vi "GUI_Cameras_v1.4.vi"() -> ()   [LabVIEW 2013]
uses:
  <vilib>/vision/NI_Vision_Development_Module.lvlib
  shared programs/MySQL/Preset Query Enum.ctl
  color tables/image color table presets.ctl
  <vilib>/Utility/miscctls.llb/LVRectTypeDef.ctl
panel:
  in  "resize":bool
  in  "Tab Control":T1(tab)
  in  "size 2":cluster{"xhair size":dbl, "xhair size 2":dbl}={"xhair size"=20.0, "xhair size 2"=20.0} {"xhair size 2" min=0.0 max=0.0; "xhair size" min=0.0 max=0.0}
  in  "Target.X":dbl caption="TargetX"
  in  "Target.Y":dbl caption="TargetY"
  in  "draw Xhair":bool
  out "Max Counts":dbl(slide) scale=0.0..256.0
  in  "triggerdelay":dbl
  in  "trigger":bool
  in  "save":bool
  in  "exposure":dbl=0.52 caption="Exposure"
  in  "gain":dbl
  in  "shotnumber":i32=354
  in  "LowPass":bool
  in  "Size & Tolerance":T2={"X Size"=5, "Y Size"=5, "% Tolerance"=100}
  in  "LowPass":bool
  in  "Color table":T3=enum."BWR enhance low"
  in  "ROI.OffsetY":dbl
  in  "ROI.OffsetX":dbl
  in  "ROI.Height":dbl
  in  "ROI.Width":dbl
  in  "MaxGUIPixel":dbl
  out "Centroid":cluster{"X Centroid":sgl, "Y Centroid":sgl} {"Y Centroid" format="%.2f"; "X Centroid" format="%.2f"}
  out "Y Resolution":i32
  out "X Resolution":i32
  out "Mean Value":sgl format="%.2f"
  out "GUIBinning":dbl
  in  "Maximize!!":bool
  in  "LogArray":bool
  in  "hide controls":bool
  in  "sat level":sgl=255.0
  in  "beep if sat.":bool
  out "Mean Value 2":sgl(graph)
  out "histogram":T4(graph)
  out "lineout":cluster{"x0":sgl, "dx":sgl, "Pixels Line":sgl[]}(graph)
  out "MaxCounts":dbl
  in  "FWHMx":dbl
  in  "FWHMy":dbl
  out "MeanCounts":dbl
  out "FWHMx (um)":dbl
  out "FWHMy (um)":dbl
  in  "SpatialCalibration":dbl
  in  "Analysis":bool
  out "analysis error":errorcluster
  out "top":i16
  out "left":i16
  out "Zoom changed":bool
  out "Zoom old":cluster{"X":sgl, "Y":sgl}
  out "ratio(h)":bool=TRUE
  out "fixsize":bool
  out "Change Ratio":cluster{"X":sgl, "Y":sgl}={"X"=1.6671598, "Y"=0.6151203}
  out "old Panel Bounds":T5={"Left"=105, "Top"=80, "Right"=781, "Bottom"=662}
  out "error (h)":bool
  in  "Main Tap":enum32{"IMAQ", "Network", "Internal", "Array"}(tab)
  out "Image (IMAQ)":T6(plugin-control)
  out "local Port":u16=65401
  out "Remote Host":string="192.168.10.157"
  out "port or service name":u16=65400
  in  "timeout ms (slow resp)":i32=500
  in  "reset":bool
  out "All Devices (h)":string[](array[string])
  out "centroidy":dbl
  out "fast ID (h)":refnum<k16>
  out "slow ID (h)":refnum<k16>
  out "error out":errorcluster
  out "connections (hidden)":variant[](array[variant])=[variant(refnum<k16> refnum), variant(refnum<k16> refnum)]
  in  "time to wait (main loop)":i32=200
  in  "time to wait (TCP)":i32=10
  out "Data String":string="exposure,0.520000\r\ntrigger,off\r\nsave,off\r\ngain,0.000000\r\n"
  in  "send":bool
  in  "localsavingpath":path
  out "centroidy":dbl
  out "Image (array)":dbl[][](graph)
  out "Device Name (h)":string="FakeCam1"
  out "stop":bool
  out "error message":string
  out "image connection":bool
  out "data connection ok":bool
  # "Crosshair"
  # "Data"
  # "Image"
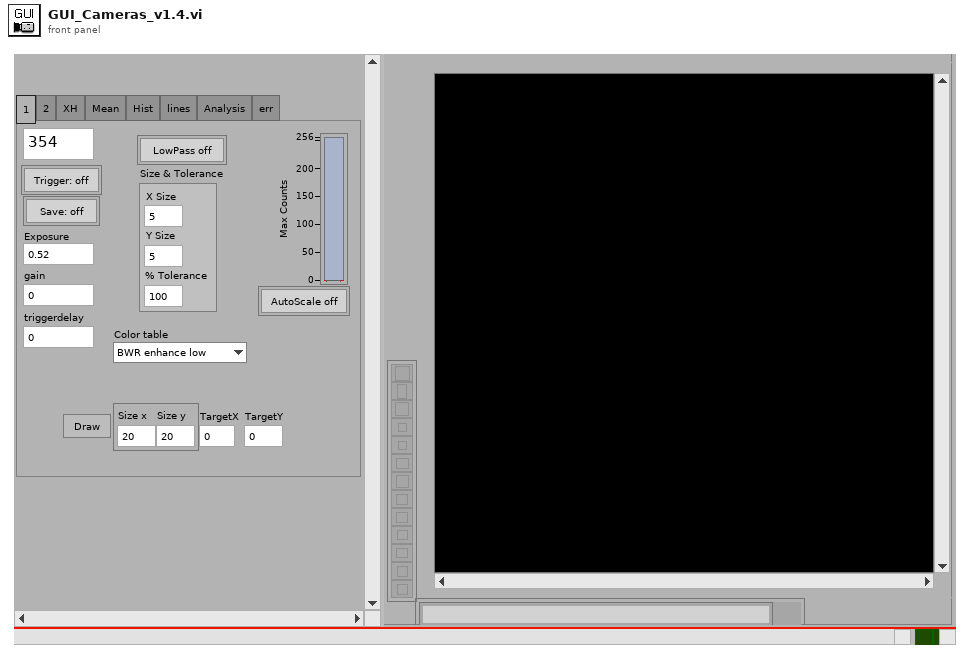
[diagram p1: front panel]
types:
  T1 = enum32{"1", "2", "XH", "Mean", "Hist", "lines", "Analysis", "err"}
  T2 = cluster{"X Size":i32, "Y Size":i32, "% Tolerance":i32}
  T3 = typedef "image color table presets.ctl" = enum16{"Greyscale", "Binary", "Gradient", "Rainbow", "Temperature", "enhance low", "blue yellow red", "BYR enhance low", "white blue yellow", "BWR enhance low", "make a new one"}
  T4 = cluster{"Starting Value":sgl, "Incremental Value":sgl, "Histogram":u32[]}
  T5 = typedef "LVRectTypeDef.ctl" = cluster{"Left":i16, "Top":i16, "Right":i16, "Bottom":i16}
  T6 = typedef "IMAQ Image.ctl" = refnum<image>
  T7 = enum16{"Grayscale", "Binary", "Gradient", "Rainbow", "Temperature", "User Defined"}
  T8 = typedef "Preset Query Enum.ctl" = enum16{"Get Locations", "Get all IPs and MACs", "Get classes", "Get expt variables to set at scanstart for particular device", "Get expt devices and variables with start values", "Get expt devices and variables (with data to get)", "Get expt devices with data to get", "Get Expt devices and GUIs", "Get all devices basic properties", "Get Virtual Devices Core Info", "Get Expt names", "Get experiment basic properties", "Get experiment alarm variables", "Get MC Ports", "Get device network comm port", "Get devicetype lvclass path", "Get basic device properties", "Get Init Order", "Get all setable variables of a device", "Get device variable aliases", "Get force values of all settable variables", "Get all variables of a devicetype", "Get all variables of a device", "Get plotter details", "Get Saved Scans", "Get Scan Info", "GetGeneralGUIs", "Get expt for plotter", "Get plotter IDs from expt", "Get all devices", "Get all Virtual Devices", "Get variable and device info for Virtual Device", "GetItemLocatorIP", "Get IPs for GUIs", "Get DeviceType from Device", "GetLocalPortRange", "GetDevicePresetVariables", "Get Device Configuration", "GetAllPresetNames", "GetAllConfigurationNames", "GetPresetDeviceNames"}
  T9 = cluster{"Left":i32, "Top":i32, "Right":i32, "Bottom":i32}
  T10 = enum32{"Invalid", "Standard", "Closed", "Hidden", "Minimized", "Maximized"}
  T11 = typedef "Image Type" = u32
  T12 = cluster{"Global Rectangle":i32[], "Contours":cluster{"Contour Type":u32, "ROI Type":u32, "Points":i32[]}[]}
  T13 = typedef "EventTypDef.ctl" = refnum<user-event>
  T14 = typedef "LVBoundsTypeDef.ctl" = cluster{"Width":u32, "Height":u32}
  T15 = typedef "ROI Descriptor" = cluster{"Global Rectangle":i32[], "Contours":cluster{"ID":enum32{"External", "Internal"}, "Type":u32, "Coordinates":i32[]}[]}
  T16 = typedef "IMAQ Line" = cluster{"Start X":i32, "Start Y":i32, "End X":i32, "End Y":i32}
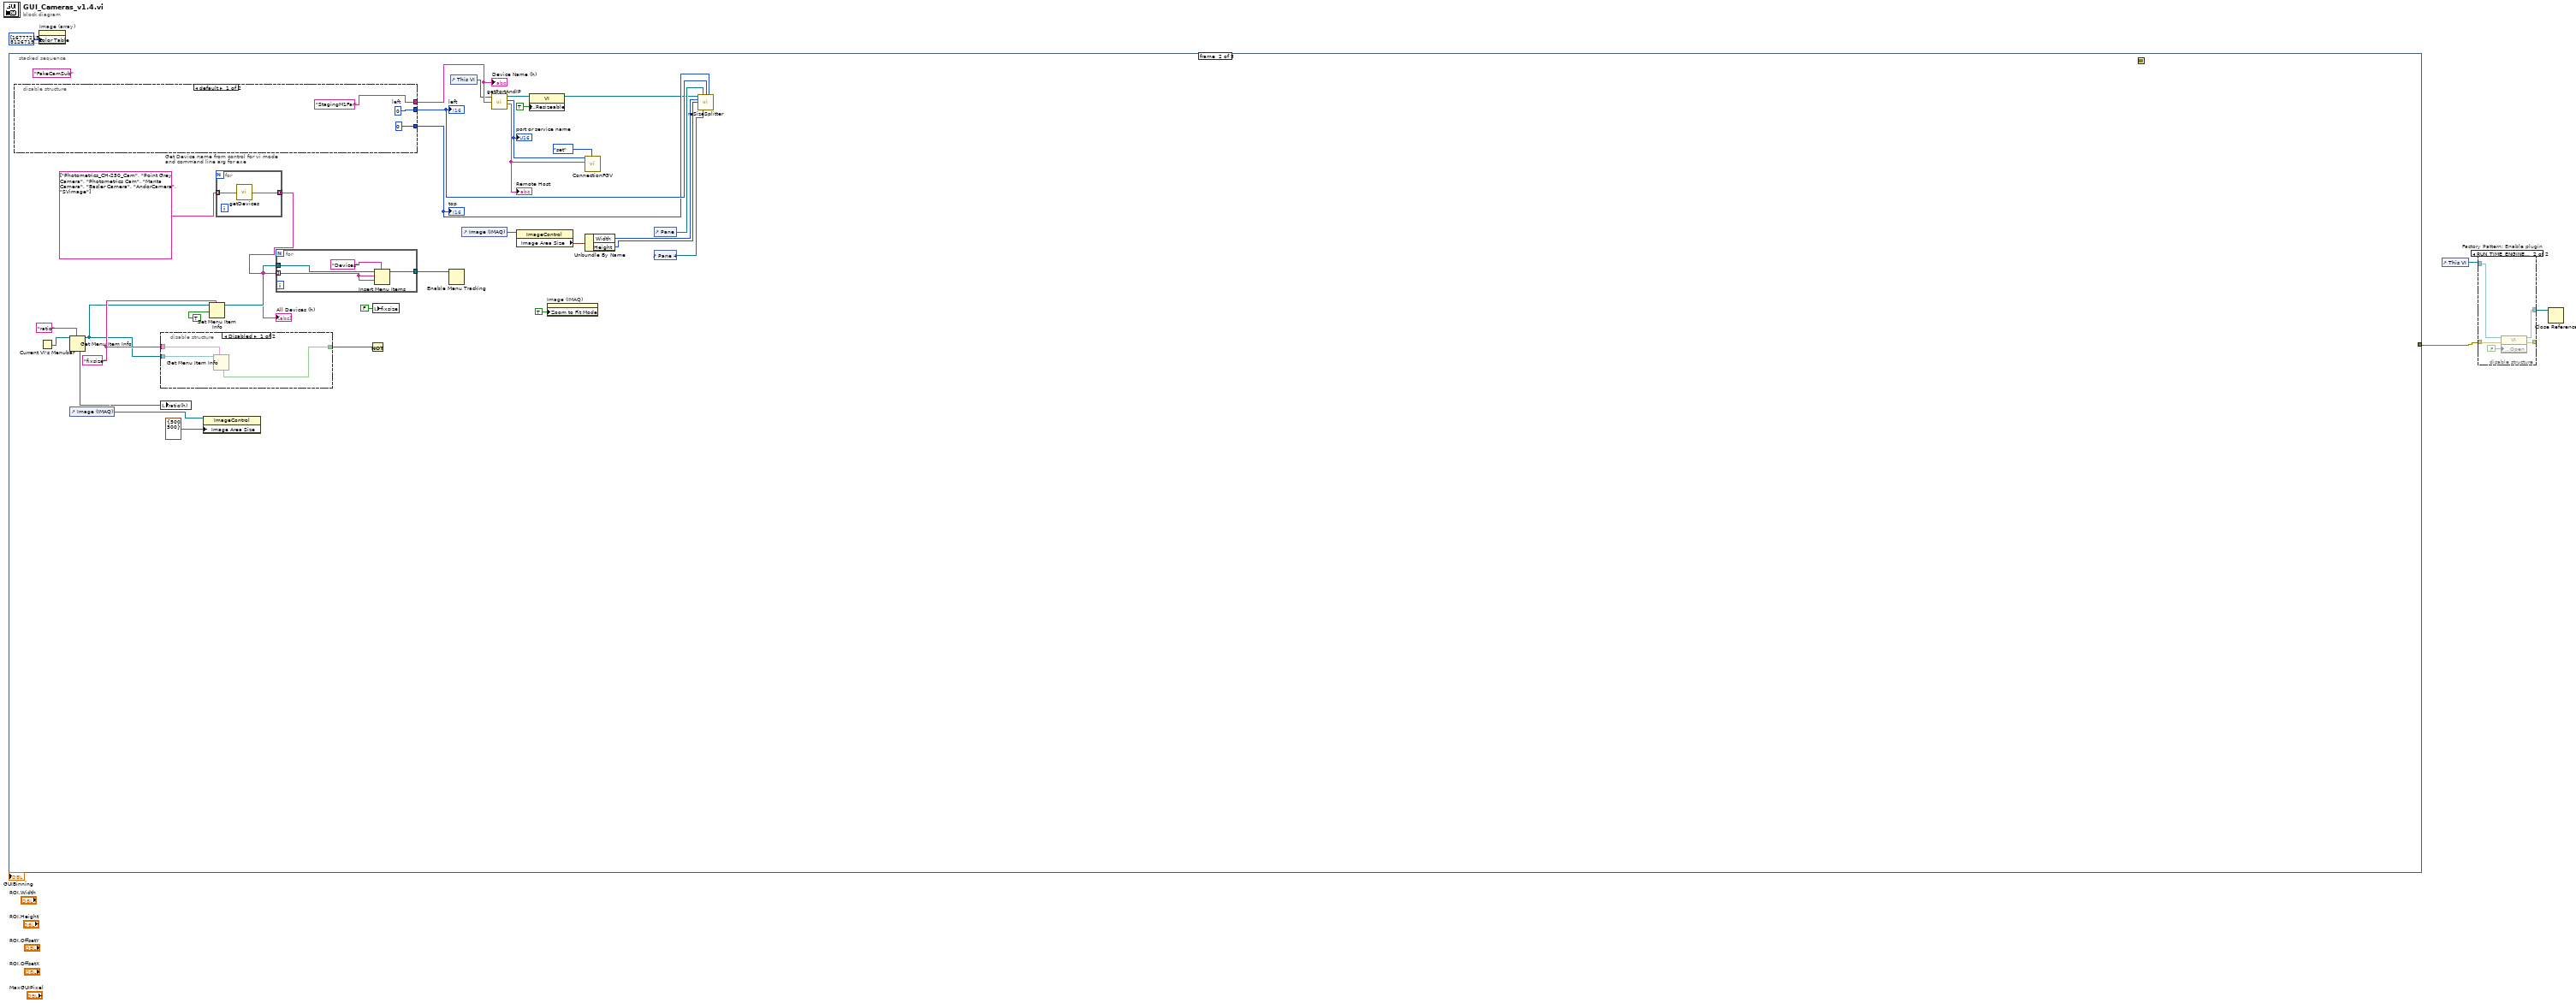
[diagram p0: block diagram]
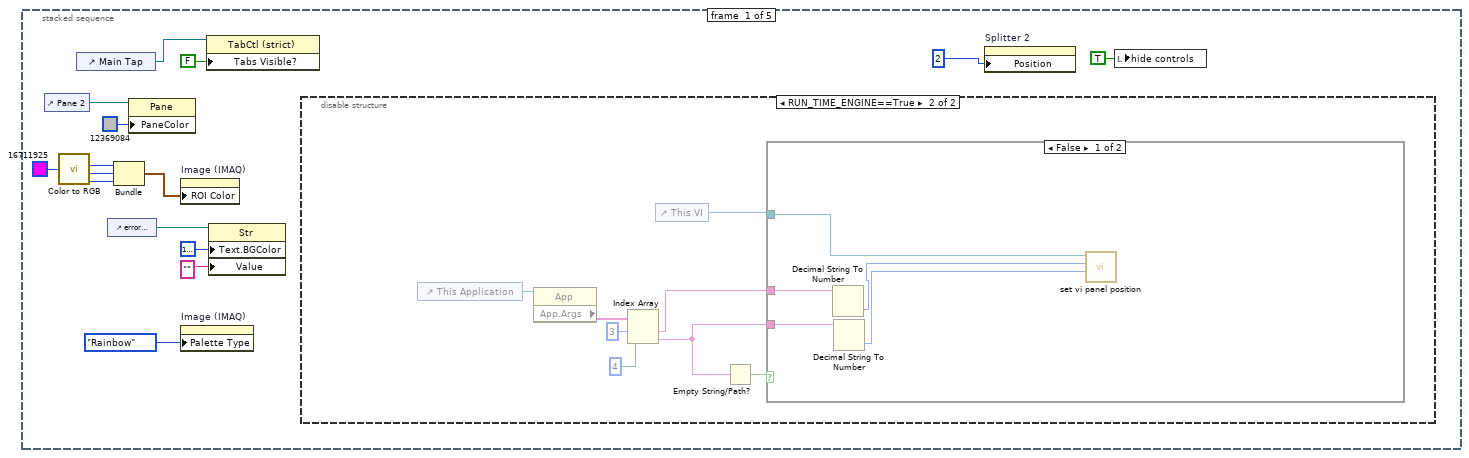
[diagram p3: hidden frame]
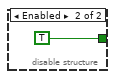
[diagram p6: hidden frame]
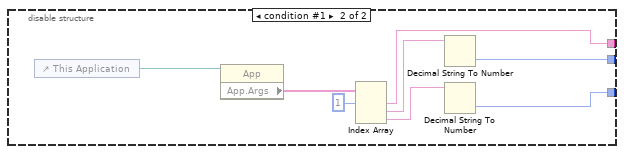
[diagram p7: hidden frame]
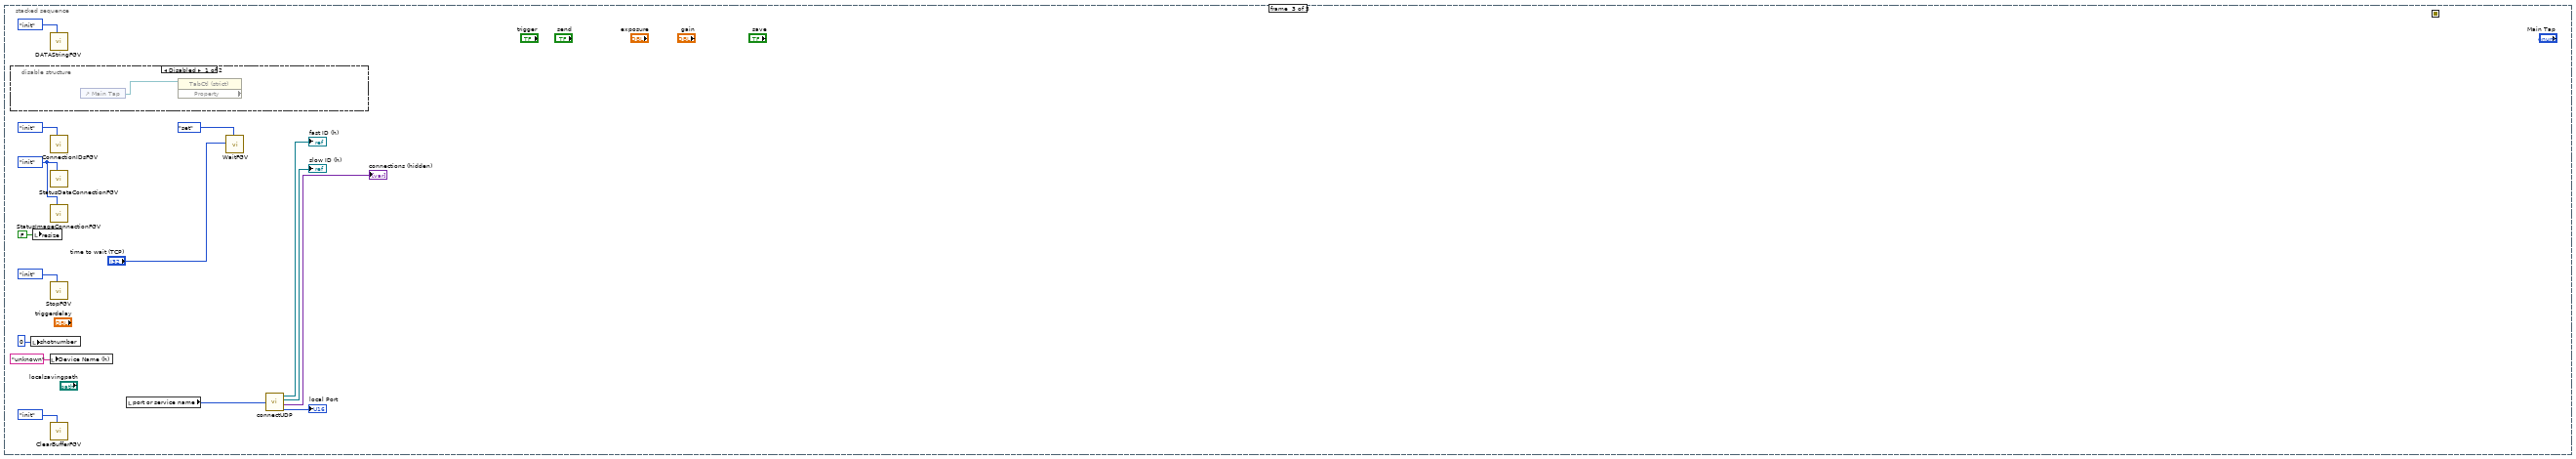
[diagram p8: hidden frame]
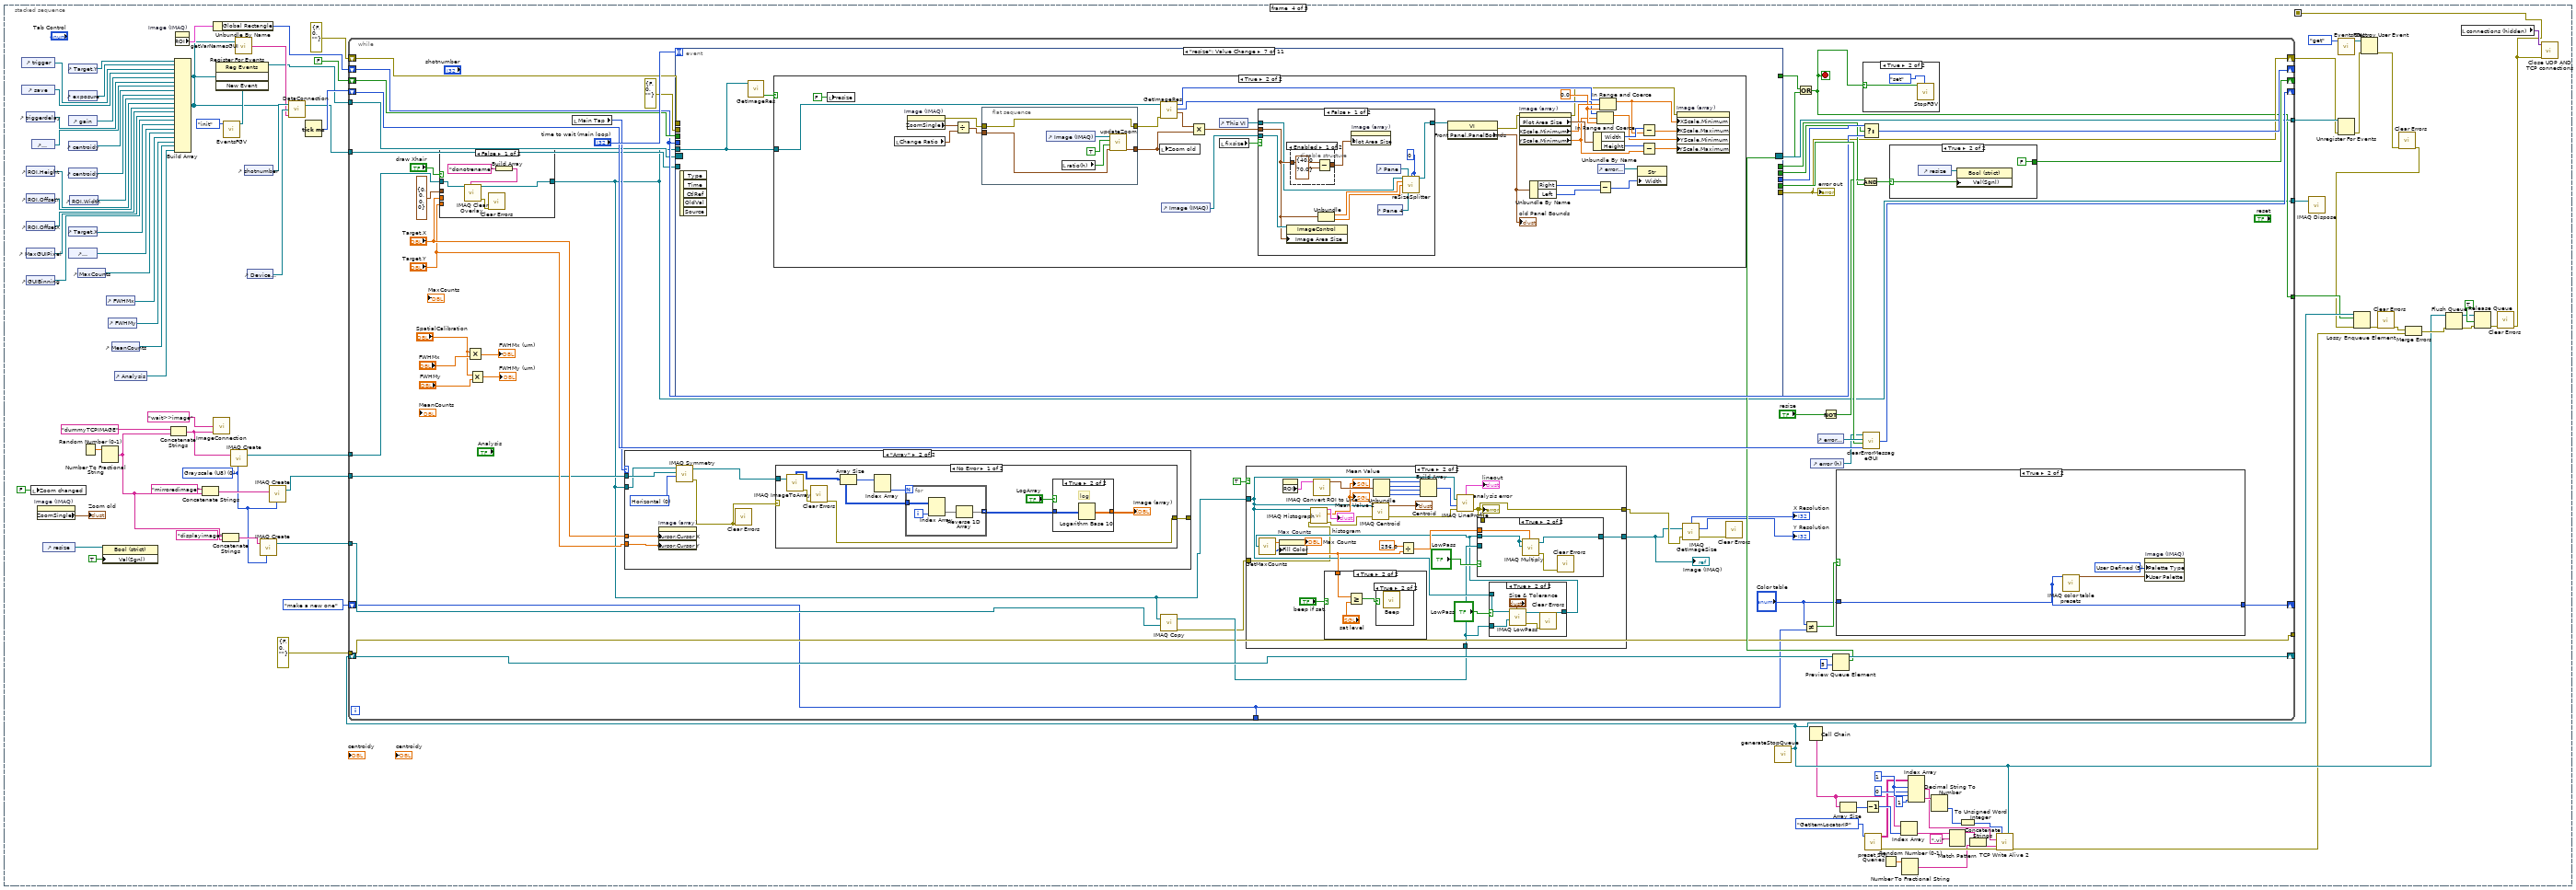
[diagram p10: hidden frame]
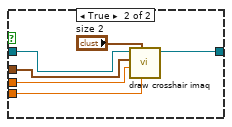
[diagram p17: hidden frame]
diagram:
  n1 = stacked-sequence {
    seq-local: [_ _ _ w135 _] -> [_ _ _ _ w558]
    tunnel: [_ _ _ _ w558] -> w2
    frame #0 {
      n2 = control-ref of="Pane 2"() -> (w14:refnum<vi>)
      n3 = call <vilib>:"Color to RGB.vi"("Color"=u32 16711925) -> ("R"=w10:u8, "G"=w9:u8, "B"=w8:u8)  [unwired: 1 out]
      n4 = control-ref of="Main Tap"() -> (w19:refnum<vi>)
      n5 = control-ref of="error message"() -> (w16:refnum<vi>)
      n6 = Bundle("R"=w10, "G"=w9, "B"=w8) -> (w7:cluster{"R":u8, "G":u8, "B":u8})  [unwired: 1 in]
      n7 = property class="Pane"(reference=w14, "PaneColor"=u32 12369084) -> ()  [unwired: 1 in, 2 out]
      n8 = property on="Image (IMAQ)" class="ImageControl"("ROI Color"=w7) -> ()  [unwired: 2 in, 2 out]
      n9 = property on="Image (IMAQ)" class="ImageControl"("Palette Type"=T7."Rainbow" ("Palette:Palette Type")) -> ()  [unwired: 2 in, 2 out]
      n10 = property class="TabCtl (strict)"(reference=w19, "Tabs Visible?"=FALSE) -> ()  [unwired: 1 in, 2 out]
      n11 = property class="Str"(reference=w16, "Text.BGColor"=u32 16777238, "Value"="") -> ()  [unwired: 1 in, 2 out]
      n12 = disable-structure shown="RUN_TIME_ENGINE==True" {
        frame condition #0 (active) {
        }
        frame condition #1 {
          n13 = control-ref of="This Application"() -> (w20:refnum<vi>)
          n14 = property class="App"(reference=w20) -> ("App.Args"=w27:string[])  [unwired: 1 in, 2 out]
          n15 = Index Array(array=w27, index #1=3 ("index"), index #2=4 ("index")) -> (element #1=w24:string, element #2=w23:string)
          n16 = control-ref of="This VI"() -> (w21:refnum<vi>)
          n17 = Empty String/Path?(string/path=w23) -> (empty?=w22:bool)
          n18 = case shown="False" w22 {
            tunnel: w24 -> [w32 _]
            tunnel: w21 -> [w28 _]
            tunnel: w23 -> [w29 _]
            frame False {
              n19 = Decimal String To Number(string=w32) -> (number=w31:i32)  [unwired: 2 in, 1 out]
              n20 = Decimal String To Number(string=w29) -> (number=w30:i32)  [unwired: 2 in, 1 out]
              n21 = call "set vi panel position.vi"("top"=w30, "left"=w31, "This VI"=w28) -> ()  [unwired: 7 in, 2 out]
            }
            frame True {
            }
          }
        }
      }
      n22 = property on="Splitter 2" class="Splitter"("Position"=2 ("Position:Left")) -> ()  [unwired: 2 in, 2 out]
      n23 = local write "hide controls"(TRUE ("hide controls")) -> ()
    }
    frame #1 {
      (unwired) "FakeCamSub" ("Device Class")
      w40 = "fixsize" ("item tag")
      n24 = disable-structure "Get Device name from control for vi mode\nand command line arg for exe" shown="default" {
        disable-tunnel: ["StagingM1Far" ("Device Name for vi mode") w81] -> w50
        disable-tunnel: [w75 w78] -> w55
        disable-tunnel: [i16 0 ("left") w77] -> w54
        frame condition #0 (active) {
          w75 = i16 0  # left
        }
        frame condition #1 {
          n25 = control-ref of="This Application"() -> (w84:refnum<vi>)
          n26 = property class="App"(reference=w84) -> ("App.Args"=w83:string[])  [unwired: 1 in, 2 out]
          n27 = Index Array(array=w83, index #1=1 ("index")) -> (element #1=w81:string, element #2=w80:string, element #3=w79:string)  [unwired: 2 in]
          n28 = Decimal String To Number(string=w80) -> (number=w78:i32)  [unwired: 2 in, 1 out]
          n29 = Decimal String To Number(string=w79) -> (number=w77:i32)  [unwired: 2 in, 1 out]
        }
      }
      "Device Name (h)" <- w50
      "left" <- w55
      "top" <- w54
      n30 = Current VI's Menubar() -> (w57:refnum<k9>)
      n31 = control-ref of="Image (IMAQ)"() -> (w43:refnum<vi>)
      n32 = Get Menu Item Info(7:"ratio" ("item tag"), 11:w57) -> (3:w39:refnum<k9>, 4:w56:bool)  [unwired: 1 in, 5 out]
      n33 = disable-structure shown="Disabled" {
        disable-tunnel: [w68 TRUE] -> w53
        disable-tunnel: w40 -> [w67 _]
        disable-tunnel: w39 -> [w66 _]
        frame Disabled {
          n34 = Get Menu Item Info(7:w67, 11:w66) -> (4:w68:bool)  [unwired: 1 in, 6 out]
        }
        frame Enabled {
        }
      }
      n35 = local write "ratio(h)"(w56) -> ()
      n36 = property class="ImageControl"(reference=w43, "Image Area Size"=cluster{"Width":u32, "Height":u32} {"Width"=500, "Height"=500} ("Image Area:Size:All Elements")) -> ()  [unwired: 1 in, 2 out]
      n37 = Set Menu Item Info(7:w40, 9:TRUE ("enabled"), 11:w39) -> (3:w38:refnum<k9>)  [unwired: 4 in, 1 out]
      n38 = for {
        tunnel: [w65] -> w34 mode=concatenating
        tunnel: string[] ["Photometrics_CH-250_Cam", "Point Grey Camera", "Photometrics Cam", "Manta Camera", "Basler Camera", "AndorCamera", "SVimage"] -> [w64] mode=indexing
        n39 = call "getDevices.vi"("Device Class"=w64) -> ("All Devices"=w65:string[])
      }
      "All Devices (h)" <- w34
      n40 = for {
        tunnel: w38 -> [w73]
        tunnel: [w72] -> w51
        tunnel: w34 -> [w70] mode=indexing
        n41 = Insert Menu Items(5:"Devices" ("menu tag"), 7:w70, 8:w70, 9:w73) -> (3:w72:refnum<k9>)  [unwired: 2 in, 2 out]
      }
      n42 = Not(x=w53) -> ()  [unwired: 1 out]
      n43 = local write "fixsize"(FALSE ("fixsize")) -> ()
      n44 = Enable Menu Tracking(4:w51) -> ()  [unwired: 2 in, 2 out]
      n45 = control-ref of="This VI"() -> (w49:refnum<vi>)
      n46 = control-ref of="Image (IMAQ)"() -> (w63:refnum<vi>)
      n47 = call "getPortAndIP.vi"("Device Name"=w50, "This Vi"=w49) -> ("Remote Host"=w44:string, "port or service name"=w45:u16, "reference out"=w48:refnum<vi>)  [unwired: 2 in, 2 out]
      "port or service name" <- w45
      "Remote Host" <- w44
      n48 = property class="ImageControl"(reference=w63) -> ("Image Area Size"=w62:cluster{"Width":u32, "Height":u32})  [unwired: 1 in, 2 out]
      n49 = property class="VI"(reference=w48, "Front Panel.Resizeable"=TRUE ("Front Panel Window:Resizable")) -> (reference out=w47:refnum<vi>)  [unwired: 1 in, 1 out]
      n50 = property on="Image (IMAQ)" class="ImageControl"("Zoom to Fit Mode"=TRUE) -> ()  [unwired: 2 in, 2 out]
      n51 = call "ConnectionFGV.vi"("command"=enum16{"get", "set", "init"}."set", "Remote Host in"=w44, "port or service name in"=w45) -> ()  [unwired: 7 in, 2 out]
      n52 = Unbundle By Name(w62) -> ("Width"=w61:u32, "Height"=w60:u32)
      n53 = control-ref of="Pane"() -> (w59:refnum<vi>)
      n54 = control-ref of="Pane 4"() -> (w52:refnum<vi>)
      n55 = call "reSizeSplitter.vi"("this vi"=w47, "pane"=w59, "left"=w55, "top"=w54, "Width"=w61, "Height"=w60, "pane2"=w52) -> ()  [unwired: 8 in, 1 out]
    }
    frame #2 {
      w95 = enum16{"get", "set", "init"}."init" ("Command")
      n56 = disable-structure shown="Disabled" {
        frame Disabled {
          n57 = control-ref of="Main Tap"() -> (w100:refnum<vi>)
          n58 = property class="TabCtl (strict)" props=[](reference=w100) -> ()  [unwired: 1 in, 3 out]
        }
        frame Enabled {
        }
      }
      n59 = local write "shotnumber"(0 ("shotnumber")) -> ()
      n60 = local write "resize"(FALSE ("resize")) -> ()
      n61 = call "DATAStringFGV.vi"("Command"=enum16{"get", "set", "init"}."init") -> ()  [unwired: 9 in, 2 out]
      n62 = call "ConnectionIDsFGV.vi"("Command"=enum16{"add", "get", "init"}."init") -> ()  [unwired: 10 in, 1 out]
      n63 = call "StatusDataConnectionFGV.vi"("Command"=w95) -> ()  [unwired: 10 in, 1 out]
      n64 = call "StatusImageConnectionFGV.vi"("Command"=w95) -> ()  [unwired: 10 in, 1 out]
      n65 = call "StopFGV.vi"("Command"=enum16{"set", "get", "init"}."init") -> ()  [unwired: 9 in, 2 out]
      n66 = local write "Device Name (h)"("unknown" ("Device Name")) -> ()
      n67 = call "ClearBufferFGV.vi"("Command"=enum16{"set", "get", "init"}."init") -> ()  [unwired: 10 in, 1 out]
      n68 = local read "port or service name"() -> (w97:u16)
      n69 = call "WaitFGV.vi"("Command"=enum16{"get", "set", "init"}."set", "milliseconds to wait"="time to wait (TCP)") -> ()  [unwired: 9 in, 1 out]
      n70 = call "connectUDP.vi"("port or service name NOT USED"=w97) -> ("fast ID (h)"=→"fast ID (h)":refnum<k16>, "slow ID (h)"=→"slow ID (h)":refnum<k16>, "connections (hidden)"=→"connections (hidden)":variant[], "local Port"=→"local Port":u16)
    }
    frame #3 {
      w124 = 1 ("index (row)")
      w101 = T11 0 items=["Grayscale (U8)", "Grayscale (I16)", "Grayscale (SGL)", "Complex (CSG)", "RGB (U32)", "HSL (U32)", "RGB (U64)", "Grayscale (U16)"] ("Image Type")
      n71 = control-ref of="trigger"() -> (w184:refnum<vi>)
      n72 = control-ref of="save"() -> (w182:refnum<vi>)
      n73 = control-ref of="triggerdelay"() -> (w180:refnum<vi>)
      n74 = control-ref of="ROI.OffsetY"() -> (w154:refnum<vi>)
      n75 = control-ref of="ROI.OffsetX"() -> (w153:refnum<vi>)
      n76 = control-ref of="MaxGUIPixel"() -> (w152:refnum<vi>)
      n77 = control-ref of="ROI.Height"() -> (w155:refnum<vi>)
      n78 = control-ref of="GUIBinning"() -> (w151:refnum<vi>)
      n79 = local write "Zoom changed"(FALSE ("Zoom changed")) -> ()
      n80 = control-ref of="localsavingpath"() -> (w176:refnum<vi>)
      n81 = property on="Image (IMAQ)" class="ImageControl"() -> ("ZoomSingle"=→"Zoom old":cluster{"X":sgl, "Y":sgl})  [unwired: 2 in, 2 out]
      n82 = control-ref of="resize"() -> (w166:refnum<vi>)
      n83 = control-ref of="Target.Y"() -> (w149:refnum<vi>)
      n84 = control-ref of="exposure"() -> (w183:refnum<vi>)
      n85 = control-ref of="gain"() -> (w181:refnum<vi>)
      n86 = control-ref of="centroidy"() -> (w175:refnum<vi>)
      n87 = control-ref of="centroidy"() -> (w169:refnum<vi>)
      n88 = control-ref of="Target.X"() -> (w150:refnum<vi>)
      n89 = control-ref of="SpatialCalibration"() -> (w148:refnum<vi>)
      n90 = control-ref of="ROI.Width"() -> (w156:refnum<vi>)
      n91 = control-ref of="MaxCounts"() -> (w147:refnum<vi>)
      n92 = Random Number (0-1)() -> (number: 0 to 1=w189:dbl)
      n93 = Number To Fractional String(number=w189) -> (F-format string=w103:string)  [unwired: 3 in]
      n94 = property class="Bool (strict)"(reference=w166, "Val(Sgnl)"=TRUE ("Value (Signaling)")) -> ()  [unwired: 1 in, 2 out]
      n95 = control-ref of="FWHMx"() -> (w146:refnum<vi>)
      n96 = control-ref of="FWHMy"() -> (w145:refnum<vi>)
      n97 = control-ref of="MeanCounts"() -> (w144:refnum<vi>)
      n98 = control-ref of="Analysis"() -> (w143:refnum<vi>)
      n99 = Concatenate Strings("dummyTCPIMAGE" ("Image Name"), w103) -> (w187:string)
      n100 = Build Array(w149, w183, w184, w182, w181, w180, w176, w175, w169, w156, w155, w154, w153, w152, w151, w150, w148, w147, w146, w145, w144, w143) -> (w163:refnum<vi>[])
      n101 = property on="Image (IMAQ)" class="ImageControl"() -> ("ROI"=w174:T12)  [unwired: 2 in, 2 out]
      n102 = Concatenate Strings("mirroredimage" ("string"), w103) -> (w108:string)
      n103 = Unbundle By Name(w174) -> ("Global Rectangle"=w173:i32[])
      n104 = call "ImageConnection.vi"("Image Name"=w187, "Image Subscriber list"="wait>>image") -> ()  [unwired: 2 in]
      n105 = Concatenate Strings("displayimage" ("string"), w103) -> (w105:string)
      n106 = call "EventsFGV.vi"("Command"=enum16{"get", "init"}."init") -> ("New Event"=w164:T13)  [unwired: 9 in, 1 out]
      n107 = register-events(w163, w164) -> (reference out=w162:refnum<event-registration>)  [unwired: 2 in, 1 out]
      n108 = call "IMAQ Create"("Image Name"=w187, "Image Type"=w101) -> ("New Image"=w190:T6)  [unwired: 3 in, 1 out]
      n109 = call "getVarNamesGUI.vi"("Array"=w163) -> ("String"=w168:string)  [unwired: 1 in]
      n110 = control-ref of="shotnumber"() -> (w171:refnum<vi>)
      n111 = control-ref of="Device Name (h)"() -> (w170:refnum<vi>)
      n112 = call "IMAQ Create"("Image Name"=w105, "Image Type"=w101) -> ("New Image"=w104:T6)  [unwired: 3 in, 1 out]
      n113 = call "IMAQ Create"("Image Name"=w108, "Image Type"=w101) -> ("New Image"=w107:T6)  [unwired: 3 in, 1 out]
      n114 = call "DataConnection.vi"("Subscriber list"=w168, "Device Name (h)"=w170, "shotnumber"=w171) -> ()
      n115 = Tick Count (ms)() -> (millisecond timer value=w177:u32)
      n116 = call "generateStopQueue.vi"() -> ("STOP Queue out"=w118:refnum<queue>)  [unwired: 10 in, 1 out]
      n117 = while {
        shift-right: [w225] -> w159
        shift-left: errorcluster {"status"=FALSE, "code"=0, "source"=""} ("error out") -> [w245]
        tunnel: w190 -> [w224]
        tunnel: [w201] -> w191
        tunnel: w163 -> [w232]
        shift-right: [w231] -> _
        shift-left: FALSE -> [w244]
        shift-right: [w243] -> _
        shift-left: w177 -> [w242]
        shift-right: [w237] -> _
        shift-left: w173 -> [w236]
        tunnel: w162 -> [w233]
        tunnel: [w226] -> w161
        tunnel: errorcluster {"status"=FALSE, "code"=0, "source"=""} ("error out") -> [w198]
        tunnel: [w198] -> _
        tunnel: [w209] -> w115
        shift-right: [w212] -> _
        shift-left: w118 -> [w213]
        tunnel: w107 -> [w207]
        tunnel: w104 -> [w200]
        shift-right: [w196] -> _
        shift-left: image_color_table_presets."make a new one" ("Color table") -> [w195]
        tunnel: [w195] -> _
        stop <- w209 stop-if-true
        n118 = case shown="False" "draw Xhair" {
          tunnel: "Target.Y" -> [_ w299]
          tunnel: "Target.X" -> [_ w300]
          tunnel: w224 -> [w297 w303]
          tunnel: [w296 w301] -> w201
          tunnel: T9 {"Left"=0, "Top"=0, "Right"=0, "Bottom"=0} ("Bounding Rectangle") -> [_ w302]
          frame False {
            n119 = Build Array("donotrename" ("String")) -> (w293:string[])
            n120 = call "IMAQ Clear Overlay"("Groups"=w293, "Image"=w297) -> ("error out"=w295:errorcluster, "Image Out"=w296:T6)  [unwired: 8 in]
            n121 = call <vilib>:"Clear Errors.vi"("error in (no error)"=w295) -> ()  [unwired: 6 in, 1 out]
          }
          frame True {
            n122 = call "draw crosshair imaq.vi"("Target.Y"=w299, "size"="size 2", "Target.X"=w300, "Bounding Rectangle"=w302, "image in"=w303) -> ("image out"=w301:T6)  [unwired: 5 in, 1 out]
          }
        }
        n123 = Multiply(x="SpatialCalibration", y="FWHMx") -> (x*y=→"FWHMx (um)":dbl)
        n124 = Multiply(x="SpatialCalibration", y="FWHMy") -> (x*y=→"FWHMy (um)":dbl)
        n125 = local read "Main Tap"() -> (w239:enum32{"IMAQ", "Network", "Internal", "Array"})
        n126 = case shown="\"Array\"" w239 {
          tunnel: w201 -> [_ w314]
          tunnel: "Target.X" -> [_ w317]
          tunnel: "Target.Y" -> [_ w316]
          tunnel: w207 -> [_ w315]
          tunnel: [_ w310] -> _
          frame "IMAQ", Default {
          }
          frame "Array" {
            w313 = u32 0 items=["Horizontal", "Vertical", "Central", "1st Diagonal", "2nd Diagonal"] ("Type of Symmetry")
            n127 = property on="Image (array)" class="IntGraph (strict)"("Cursor.Cursor X"=w317, "Cursor.Cursor Y"=w316) -> ()  [unwired: 2 in, 2 out]
            n128 = call "IMAQ Symmetry"("Type of Symmetry"=w313, "Image Dst"=w315, "Image Src"=w314) -> ("error out"=w311:errorcluster, "Image Dst Out"=w312:T6)  [unwired: 2 in]
            n129 = call <vilib>:"Clear Errors.vi"("error in (no error)"=w311) -> ()  [unwired: 6 in, 1 out]
            n130 = case shown="No Error" w311 {
              tunnel: w312 -> [w320 _]
              tunnel: [w319 _] -> w310
              frame No Error {
                n131 = call "IMAQ ImageToArray"("Image"=w320) -> ("error out"=w326:errorcluster, "Image Pixels (U8)"=w318:u8[][])  [unwired: 3 in, 3 out]
                n132 = call <vilib>:"Clear Errors.vi"("error in (no error)"=w326) -> ("error out"=w319:errorcluster)  [unwired: 6 in]
                n133 = Array Size(array=w318) -> (size(s)=w325:i32[])
                n134 = Index Array(array=w325) -> (element #2=w324:i32)  [unwired: 2 in, 1 out]
                n135 = for {
                  N: w324 -> [_]
                  tunnel: w318 -> [w333]
                  tunnel: [w331] -> w322 mode=indexing
                  i -> [w330]
                  n136 = Index Array(array=w333, index (col)=w330) -> (element=w332:u8[])  [unwired: 1 in]
                  n137 = Reverse 1D Array(array=w332) -> (reversed array=w331:u8[])
                }
                n138 = case shown="True" "LogArray" {
                  tunnel: w322 -> [w327 w329]
                  tunnel: [w327 w328] -> w321
                  frame False {
                  }
                  frame True {
                    # "log"
                    n139 = Logarithm Base 10(1:w329) -> (0:w328:dbl[][])
                  }
                }
                "Image (array)" <- w321
              }
              frame Error {
              }
            }
          }
        }
        n140 = event shown="[6] \"resize\": Value Change" {
          selector: w233 -> [_ _ _ _ _ _ _ _ _ _ _]
          dyn-events: [_ _ _ _ _ _ _ _ _ _ _] -> w226
          timeout: "time to wait (main loop)" -> [_ _ _ _ _ _ _ _ _ _ _]
          tunnel: [w339 _ _ _ _ _ _ w457 _ _ _] -> w225
          tunnel: errorcluster {"status"=FALSE, "code"=0, "source"=""} ("error out") -> [w341 _ _ _ _ _ _ _ _ _ _]
          tunnel: w245 -> [_ _ _ _ _ _ _ w457 _ _ _]
          tunnel: [TRUE _ _ _ _ _ _ _ _ _ _] -> w240
          tunnel: [_ _ _ _ _ _ _ _ w460 _ _] -> w211
          tunnel: w244 -> [_ _ _ _ _ _ _ _ _ _ _]
          tunnel: [_ w349 w361 TRUE _ _ _ _ _ _ _] -> w228
          tunnel: [_ _ _ _ _ _ _ _ _ _ w534] -> w238
          tunnel: w236 -> [_ _ _ _ _ _ _ _ _ _ w535]
          tunnel: [_ _ _ _ _ _ _ _ _ _ w533] -> w235
          tunnel: w201 -> [_ _ _ _ _ _ w401 _ _ _ w536]
          tunnel: w232 -> [_ _ _ _ _ w391 _ _ _ _ _]
          event Value Change {
            n141 = event-data() -> ("CtlRef"=w336:refnum<vi>, "NewVal"=w335:variant)  [unwired: 1 in, 3 out]
            n142 = call "SendCommandEvent.vi"("timeout ms (slow resp)"="timeout ms (slow resp)", "error out 2"=w341, "NewVal"=w335, "CtlRef"=w336) -> ("error out"=w339:errorcluster, "error (h)"=→"error (h)":bool, "error message"=→"error message":string)  [unwired: 4 in, 1 out]
          }
          event Panel Resize {
            n143 = event-data() -> ("Time"=w347:u32, "OldBnds"=w344:T5, "NewBnds"=w343:T5)  [unwired: 1 in, 4 out]
            n144 = Tick Count (ms)() -> (millisecond timer value=w348:u32)
            n145 = Subtract(x=w348, y=w347) -> (x-y=w346:u32)
            n146 = Equal?(x=w344, y=w343) -> (x = y?=w342:bool)
            n147 = Greater?(x=w346, y=u32 1000) -> ()  [unwired: 1 out]
            n148 = case shown="True" w342 {
              tunnel: w343 -> [w355 _]
              tunnel: [TRUE _] -> w349
              tunnel: w344 -> [_ _]
              frame True {
                n149 = local read "old Panel Bounds"() -> (w350:T5)
                n150 = call "getWidthAndHight.vi"("OldBnds"=w350) -> ("output cluster"=w353:cluster{"X":sgl, "Y":sgl})
                n151 = call "getWidthAndHight.vi"("OldBnds"=w355) -> ("output cluster"=w352:cluster{"X":sgl, "Y":sgl})
                n152 = Divide(x=w353, y=w352) -> (x/y=→"Change Ratio":cluster{"X":sgl, "Y":sgl})
              }
              frame False {
              }
            }
          }
          event "Maximize!!": Value Change {
            n153 = event-data() -> ()  [unwired: 1 in, 5 out]
            n154 = property class="VI"() -> (error out=w356:errorcluster, "Front Panel.PanelBounds"=w357:T5)  [unwired: 2 in, 1 out]
            n155 = case shown="True" "Maximize!!" {
              tunnel: w357 -> [w371 w375]
              tunnel: [w371 w375] -> w359
              tunnel: [_ w374] -> w358
              tunnel: w356 -> [_ w372]
              frame False {
              }
              frame True {
                n156 = local write "Maximize!!"(FALSE ("Maximize!!")) -> ()
                n157 = property class="VI"(error in=w372, "Front Panel Window:State"=T10."Maximized") -> (error out=w374:errorcluster)  [unwired: 1 in, 1 out]
                n158 = Wait (ms)(milliseconds to wait=u32 200) -> ()  [unwired: 1 out]
              }
            }
            n159 = case shown="True" TRUE {
              tunnel: [TRUE _] -> w361
              tunnel: w359 -> [w367 _]
              tunnel: w358 -> [w365 _]
              frame True {
                n160 = property class="VI"(error in=w365) -> ("Front Panel.PanelBounds"=w366:T5)  [unwired: 1 in, 2 out]
                n161 = call "getWidthAndHight.vi"("OldBnds"=w367) -> ("output cluster"=w370:cluster{"X":sgl, "Y":sgl})
                n162 = call "getWidthAndHight.vi"("OldBnds"=w366) -> ("output cluster"=w369:cluster{"X":sgl, "Y":sgl})
                n163 = Divide(x=w370, y=w369) -> (x/y=w363:cluster{"X":sgl, "Y":sgl})
                n164 = local write "Change Ratio"(w363) -> ()
                n165 = local write "resize"(TRUE ("resize")) -> ()
              }
              frame False {
              }
            }
          }
          event "hide controls": Value Change {
            n166 = event-data() -> ("NewVal"=w381:bool)  [unwired: 1 in, 4 out]
            n167 = case shown="True" w381 {
              tunnel: [367 ("Position:Left") 2 ("Position:Left")] -> w380
              frame False {
              }
              frame True {
              }
            }
            n168 = local write "Change Ratio"(cluster{"X":sgl, "Y":sgl} {"X"=1.0, "Y"=1.0} ("Change Ratio")) -> ()
            n169 = property on="Splitter 2" class="Splitter"("Position"=w380) -> ()  [unwired: 2 in, 2 out]
          }
          event "reset": Value Change {
            n170 = event-data() -> ()  [unwired: 1 in, 5 out]
            n171 = flat-sequence {
              frame #0 {
                n172 = local read "connections (hidden)"() -> (w385:variant[])
                n173 = call "Close UDP AND TCP connections.vi"("appended array"=w385) -> ()  [unwired: 7 in]
              }
              frame #1 {
                n174 = call "ConnectionFGV.vi"("command"=enum16{"get", "set", "init"}."get") -> ("port or service name out"=w387:u16)  [unwired: 9 in, 1 out]
                n175 = call "connectUDP.vi"("port or service name NOT USED"=w387) -> ("connections (hidden)"=w386:variant[])  [unwired: 3 out]
                n176 = local write "connections (hidden)"(w386) -> ()
              }
              frame #2 {
                n177 = Wait (ms)(milliseconds to wait=u32 500) -> ()  [unwired: 1 out]
              }
              frame #3 {
                n178 = property on="Image (IMAQ)" class="ImageControl"("Zoom to Fit Mode"=TRUE) -> ()  [unwired: 2 in, 2 out]
              }
            }
            n179 = local write "reset"(FALSE ("reset")) -> ()
          }
          event User Event {
            n180 = event-data() -> ("EventEnum"=w392:enum16{"new data", "connection status update"})  [unwired: 1 in, 3 out]
            n181 = case shown="\"new data\", Default" w392 {
              tunnel: w391 -> [w394 _]
              frame "new data", Default {
                n182 = call "DATAStringFGV.vi"("Command"=enum16{"get", "set", "init"}."get") -> ("Data String out"=w393:string)  [unwired: 9 in, 1 out]
                "Data String" <- w393
                n183 = call "Update Indicators (Data String to ref array).vi"("Array"=w394, "Data String"=w393) -> ()  [unwired: 12 in, 2 out]
              }
              frame "connection status update" {
                n184 = call "StatusDataConnectionFGV.vi"("Command"=enum16{"get", "set", "init"}."get") -> ("Data Connection out"=→"image connection":bool)  [unwired: 10 in]
                n185 = call "StatusImageConnectionFGV.vi"("Command"=enum16{"get", "set", "init"}."get") -> ("Image Connection out"=→"data connection ok":bool)  [unwired: 10 in]
              }
            }
          }
          event "resize": Value Change {
            n186 = event-data() -> ()  [unwired: 1 in, 5 out]
            n187 = call "GetImageRes.vi"("Image"=w401) -> ("valid Image"=w400:bool)  [unwired: 6 in, 4 out]
            n188 = case shown="True" w400 {
              tunnel: w401 -> [_ w410]
              frame False {
                n189 = local write "resize"(FALSE ("resize")) -> ()
              }
              frame True {
                w418 = 0.0 ("lower limit")
                n190 = local write "resize"(FALSE ("resize")) -> ()
                n191 = local read "Change Ratio"() -> (w434:cluster{"X":sgl, "Y":sgl})
                n192 = property on="Image (IMAQ)" class="ImageControl"() -> (error out=w405:errorcluster, "ZoomSingle"=w435:cluster{"X":sgl, "Y":sgl})  [unwired: 2 in, 1 out]
                n193 = Divide(x=w435, y=w434) -> (x/y=w404:cluster{"X":sgl, "Y":sgl})
                n194 = flat-sequence {
                  tunnel: [w439] -> w403
                  tunnel: w404 -> [w437]
                  tunnel: [w436] -> w406
                  tunnel: w405 -> [w436]
                  frame #0 {
                    n195 = control-ref of="Image (IMAQ)"() -> (w441:refnum<vi>)
                    n196 = local read "ratio(h)"() -> (w440:bool)
                    n197 = call "updateZoom.vi"("Zoom old"=w437, "ratio(h)"=w440, "update Zoom"=TRUE, "imageRef"=w441) -> ("Zoom out"=w439:cluster{"X":sgl, "Y":sgl})  [unwired: 7 in]
                  }
                }
                n198 = local write "Zoom old"(w403) -> ()
                n199 = call "GetImageRes.vi"("error in (no error)"=w406, "Image"=w410) -> ("Image Area:Size:All Elements"=w411:cluster{"Width":u32, "Height":u32}, "Y Resolution"=w412:i32, "X Resolution"=w413:i32)  [unwired: 5 in, 2 out]
                n200 = control-ref of="Image (IMAQ)"() -> (w425:refnum<vi>)
                n201 = Multiply(x=w411, y=w403) -> (x*y=w433:cluster{sgl, sgl})
                n202 = control-ref of="This VI"() -> (w414:refnum<vi>)
                n203 = local read "fixsize"() -> (w426:bool)
                n204 = case shown="False" w426 {
                  tunnel: w433 -> [w445 _]
                  tunnel: w414 -> [w442 w456]
                  tunnel: [w448 w456] -> w431
                  tunnel: w425 -> [w447 _]
                  frame False {
                    w443 = i16 0 ("left")
                    n205 = property class="ImageControl"(reference=w447, "Image Area Size"=w445) -> ()  [unwired: 1 in, 2 out]
                    n206 = disable-structure shown="Enabled" {
                      disable-tunnel: w445 -> [w454 w455]
                      disable-tunnel: [w453 w455] -> w444
                      frame Enabled {
                        n207 = Subtract(x=w454, y=cluster{sgl, sgl} {40.0, 70.0}) -> (x-y=w453:cluster{sgl, sgl})
                      }
                      frame Disabled {
                      }
                    }
                    n208 = Unbundle(w445) -> (w450:sgl, w451:sgl)
                    n209 = property on="Image (array)" class="IntGraph (strict)"("Plot Area Size"=w444) -> ()  [unwired: 2 in, 2 out]
                    n210 = control-ref of="Pane"() -> (w449:refnum<vi>)
                    n211 = control-ref of="Pane 4"() -> (w446:refnum<vi>)
                    n212 = call "reSizeSplitter.vi"("this vi"=w442, "pane"=w449, "left"=w443, "top"=w443, "Width"=w450, "Height"=w451, "pane2"=w446) -> ("reference out"=w448:refnum<vi>)  [unwired: 8 in]
                  }
                  frame True {
                  }
                }
                n213 = property class="VI"(reference=w431) -> (error out=w409:errorcluster, "Front Panel.PanelBounds"=w430:T5)  [unwired: 1 in, 1 out]
                "old Panel Bounds" <- w430
                n214 = property on="Image (array)" class="IntGraph (strict)"(error in=w409) -> (error out=w408:errorcluster, "Plot Area Size"=w424:T14, "XScale.Minimum"=w419:dbl, "YScale.Minimum"=w417:dbl)  [unwired: 1 in, 1 out]
                n215 = Unbundle By Name(w430) -> ("Right"=w429:i16, "Left"=w428:i16)
                n216 = Unbundle By Name(w424) -> ("Width"=w423:u32, "Height"=w421:u32)
                n217 = In Range and Coerce(upper limit=w412, x=w417, lower limit=w418) -> (coerced(x)=w416:dbl)  [unwired: 1 out]
                n218 = Subtract(x=w429, y=w428) -> (x-y=w427:i16)
                n219 = control-ref of="error message"() -> (w432:refnum<vi>)
                n220 = In Range and Coerce(upper limit=w413, x=w419, lower limit=w418) -> (coerced(x)=w420:dbl)  [unwired: 1 out]
                n221 = property class="Str"(reference=w432, "Width"=w427) -> ()  [unwired: 1 in, 2 out]
                n222 = Subtract(x=w423, y=w420) -> (x-y=w422:dbl)
                n223 = Subtract(x=w421, y=w417) -> (x-y=w415:dbl)
                n224 = property on="Image (array)" class="IntGraph (strict)"(error in=w408, "XScale.Minimum"=w420, "XScale.Maximum"=w422, "YScale.Minimum"=w416, "YScale.Maximum"=w415) -> ()  [unwired: 1 in, 2 out]
              }
            }
          }
          event Timeout {
            n225 = event-data() -> ()  [unwired: 1 in, 2 out]
          }
          event Menu Selection (User) {
            n226 = event-data() -> ("MenuRef"=w459:refnum<k9>, "ItemTag"=w458:string)  [unwired: 1 in, 3 out]
            n227 = case shown="\"Controls\"" w458 {
              tunnel: [_ w466] -> w460
              tunnel: w458 -> [_ w464]
              tunnel: w459 -> [_ w463]
              frame "Controls" {
                n228 = local read "hide controls"() -> (w462:bool)
                n229 = Not(x=w462) -> (.not. x?=w461:bool)
                n230 = property on="hide controls" class="Bool (strict)"("Val(Sgnl)"=w461) -> ()  [unwired: 2 in, 2 out]
              }
              frame Default {
                n231 = Equal?(x="Exit", y=w464) -> (x = y?=w466:bool)
                "stop" <- w466
                n232 = property on="Main Tap" class="TabCtl (strict)"() -> ("Value"=w468:enum32{"IMAQ", "Network", "Internal", "Array"})  [unwired: 2 in, 2 out]
                n233 = case shown="False" w466 {
                  tunnel: w468 -> [w527 _]
                  tunnel: w464 -> [w526 _]
                  tunnel: [w523 errorcluster {"status"=FALSE, "code"=0, "source"=""} ("error out")] -> w465
                  frame False {
                    n234 = call <userlib>:"Set Enum String Value__ogtk.vi"("String Value"=w526, "Default Enum Value"=w527) -> ("error out"=w525:errorcluster, "Enum"=w529:variant)  [unwired: 8 in]
                    n235 = Variant To Data(error in=w525, type=w527, Variant=w529) -> (data=w528:enum32{"IMAQ", "Network", "Internal", "Array"}, error out=w524:errorcluster)
                    n236 = property on="Main Tap" class="TabCtl (strict)"(error in=w524, "Value"=w528) -> (error out=w523:errorcluster)  [unwired: 1 in, 1 out]
                  }
                  frame True {
                  }
                }
                n237 = case shown="Error" w465 {
                  tunnel: w463 -> [_ w472]
                  tunnel: w464 -> [_ w476]
                  tunnel: [_ w477] -> _
                  frame No Error {
                  }
                  frame Error {
                    n238 = local read "All Devices (h)"() -> (w474:string[])
                    n239 = Search 1D Array(1D array=w474, element=w476) -> (index of element=w475:i32)  [unwired: 1 in]
                    n240 = Get Menu Item Info(7:w476, 11:w472) -> (0:w473:errorcluster, 2:w479:string, 4:w480:bool)  [unwired: 1 in, 4 out]
                    n241 = Not(x=w480) -> (.not. x?=w478:bool)
                    n242 = Greater Or Equal To 0?(x=w475) -> (x >= 0?=w471:bool)
                    n243 = case shown="True" w471 {
                      tunnel: w474 -> [_ w484]
                      tunnel: w473 -> [_ _]
                      tunnel: w472 -> [w481 w483]
                      tunnel: [w481 w482] -> w470
                      frame False {
                      }
                      frame True {
                        n244 = for {
                          tunnel: w484 -> [w488] mode=indexing
                          tunnel: w483 -> [w486]
                          tunnel: [w485] -> w482
                          n245 = Set Menu Item Info(6:FALSE ("checked"), 7:w488, 11:w486) -> (3:w485:refnum<k9>)  [unwired: 4 in, 1 out]
                        }
                      }
                    }
                    n246 = case shown="Default" w476 {
                      selector: w476 -> [_ w494 _ _ w515 _ _]
                      tunnel: w478 -> [w489 w492 w505 _ _ _ w520]
                      tunnel: [_ _ TRUE _ _ _ _] -> w477
                      tunnel: w471 -> [_ w495 _ _ _ _ _]
                      tunnel: [w489 w493 w505 _ _ _ w520] -> w469
                      frame "fixsize" {
                        n247 = Not(x=w489) -> (.not. x?=w490:bool)
                        n248 = control-ref of="This VI"() -> (w491:refnum<vi>)
                        n249 = property class="VI"(reference=w491, "Front Panel.Resizeable"=w490) -> ()  [unwired: 1 in, 2 out]
                        "fixsize" <- w489
                      }
                      frame Default {
                        n250 = case shown="True" w495 {
                          tunnel: w494 -> [_ w503]
                          tunnel: [_ w499] -> w493
                          tunnel: w492 -> [_ w499]
                          frame False {
                          }
                          frame True {
                            n251 = control-ref of="This VI"() -> (w502:refnum<vi>)
                            n252 = control-ref of="reset"() -> (w501:refnum<vi>)
                            n253 = call "getPortAndIP.vi"("Device Name"=w503, "This Vi"=w502) -> ("Remote Host"=w496:string, "port or service name"=w497:u16)  [unwired: 2 in, 3 out]
                            n254 = local write "port or service name"(w497) -> ()
                            n255 = local write "Remote Host"(w496) -> ()
                            n256 = property class="Bool (strict)"(reference=w501, "Val(Sgnl)"=TRUE ("Value (Signaling)")) -> ()  [unwired: 1 in, 2 out]
                            n257 = call "ConnectionFGV.vi"("command"=enum16{"get", "set", "init"}."set", "Remote Host in"=w496, "port or service name in"=w497) -> ()  [unwired: 7 in, 2 out]
                          }
                        }
                      }
                      frame "ratio" {
                        n258 = property on="Image (IMAQ)" class="ImageControl"() -> ("ZoomSingle"=w504:cluster{"X":sgl, "Y":sgl})  [unwired: 2 in, 2 out]
                        n259 = local write "Zoom old"(w504) -> ()
                        "ratio(h)" <- w505
                      }
                      frame "Local Saving Path" {
                        n260 = control-ref of="localsavingpath"() -> (w507:refnum<vi>)
                        n261 = property class="Path"(reference=w507) -> (reference out=w510:refnum<vi>, "Value"=w511:path)  [unwired: 1 in, 1 out]
                        n262 = call "changePath.vi"("Local Saving in (h)"=w511) -> ("change (h)"=w509:bool, "Local Saving out (h)"=w508:path)  [unwired: 9 in]
                        n263 = case shown="True" w509 {
                          tunnel: w510 -> [_ w513]
                          tunnel: w508 -> [_ w512]
                          frame False {
                          }
                          frame True {
                            n264 = property class="Path"(reference=w513, "Val(Sgnl)"=w512) -> ()  [unwired: 1 in, 2 out]
                          }
                        }
                      }
                      frame "Binary", "Gradient", "Grayscale", "Rainbow", "Temperature" {
                        n265 = Scan From String(input string=w515, default 1=T7."Grayscale" ("Palette:Palette Type")) -> (output 1=w514:T7)  [unwired: 3 in, 3 out]
                        n266 = property on="Image (IMAQ)" class="ImageControl"("Palette Type"=w514) -> ()  [unwired: 2 in, 2 out]
                      }
                      frame "reset" {
                        n267 = control-ref of="reset"() -> (w518:refnum<vi>)
                        n268 = property class="Bool (strict)"(reference=w518, "Val(Sgnl)"=TRUE ("Value (Signaling)")) -> ()  [unwired: 1 in, 2 out]
                      }
                      frame "clear" {
                        n269 = control-ref of="reset"() -> (w522:refnum<vi>)
                        n270 = call "ClearBufferFGV.vi"("Command"=enum16{"set", "get", "init"}."set", "clear buffer"=w520) -> ()  [unwired: 9 in, 1 out]
                        n271 = property class="Bool (strict)"(reference=w522, "Val(Sgnl)"=TRUE ("Value (Signaling)")) -> ()  [unwired: 1 in, 2 out]
                      }
                    }
                    n272 = Set Menu Item Info(6:w469, 7:w476, 10:w479, 11:w470) -> ()  [unwired: 3 in, 2 out]
                  }
                }
              }
            }
          }
          event "time to wait (TCP)": Value Change {
            n273 = event-data() -> ("NewVal"=w532:i32)  [unwired: 1 in, 4 out]
            n274 = call "WaitFGV.vi"("Command"=enum16{"get", "set", "init"}."set", "milliseconds to wait"=w532) -> ()  [unwired: 9 in, 1 out]
          }
          event "Image (IMAQ)": Mouse Up {
            n275 = event-data() -> ()  [unwired: 1 in, 5 out]
            n276 = disable-structure shown="Disabled" {
              disable-tunnel: w536 -> [w551 _]
              disable-tunnel: w535 -> [w549 _]
              disable-tunnel: [w548 _] -> w534
              disable-tunnel: [w542 _] -> w533
              frame Disabled {
                n277 = local read "Zoom old"() -> (w539:cluster{"X":sgl, "Y":sgl})
                n278 = property on="Image (IMAQ)" class="ImageControl"() -> ("ZoomSingle"=w538:cluster{"X":sgl, "Y":sgl})  [unwired: 2 in, 2 out]
                n279 = property on="Image (IMAQ)" class="ImageControl"() -> ("ROI"=w550:T12)  [unwired: 2 in, 2 out]
                n280 = Unbundle By Name(w550) -> ("Global Rectangle"=w548:i32[])
                n281 = Unbundle By Name(w538) -> ("X"=w540:sgl)
                n282 = Unbundle By Name(w539) -> ("X"=w541:sgl)
                n283 = Not Equal?(x=w549, y=w548) -> (x != y?=w552:bool[])
                n284 = Empty Array?(array=w548) -> (empty?=w547:bool)
                n285 = Not Equal?(x=w540, y=w541) -> (x != y?=w537:bool)
                "Zoom changed" <- w537
                n286 = Empty Array?(array=w549) -> (empty?=w545:bool)
                n287 = Or Array Elements(Boolean array=w552) -> (logical OR=w543:bool)
                n288 = Not(x=w547) -> (.not. x?=w546:bool)
                n289 = case shown="True" w537 {
                  tunnel: w538 -> [_ w555]
                  frame False {
                  }
                  frame True {
                    n290 = local write "Zoom old"(w555) -> ()
                  }
                }
                n291 = case shown="True" w537 {
                  selector: w537 -> [_ w553]
                  frame False {
                  }
                  frame True {
                    n292 = control-ref of="resize"() -> (w554:refnum<vi>)
                    n293 = property class="Bool (strict)"(reference=w554, "Val(Sgnl)"=w553) -> ()  [unwired: 1 in, 2 out]
                  }
                }
                n294 = And(x=w545, y=w546) -> (x .and. y?=w544:bool)
                n295 = Or(x=w543, y=w544) -> (x .or. y?=w542:bool)
                n296 = case shown="True" w542 {
                  tunnel: w551 -> [_ _]
                  tunnel: w550 -> [_ w557]
                  frame False {
                  }
                  frame True {
                    n297 = call "ROI thickener.vi"("ROI Descriptor in"=w557) -> ("ROI Descriptor out"=w556:T15)  [unwired: 1 in, 1 out]
                    n298 = property on="Image (IMAQ)" class="ImageControl"("ROI"=w556) -> ()  [unwired: 2 in, 2 out]
                  }
                }
              }
              frame Enabled {
              }
            }
          }
        }
        "error out" <- w225
        n299 = call "IMAQ Copy"("Image Dst"=w200, "Image Src"=w201) -> ("error out"=w197:errorcluster, "Image Dst Out"=w199:T6)  [unwired: 4 in]
        n300 = case shown="True" TRUE ("localanalysis") {
          tunnel: w201 -> [w252 w256]
          tunnel: [_ w263] -> w203
          tunnel: [w252 w257] -> w202
          tunnel: w199 -> [_ w255]
          tunnel: w197 -> [_ w253]
          frame False {
          }
          frame True {
            n301 = property on="Image (IMAQ)" class="ImageControl"() -> ("ROI"=w275:T12)  [unwired: 2 in, 2 out]
            n302 = call "IMAQ Histograph"("error in (no error)"=w253, "Image"=w256) -> ("error out"=w267:errorcluster, "Mean Value"=→"Mean Value" →"Mean Value 2":sgl, "Histogram Graph"=→"histogram":T4)  [unwired: 6 in, 1 out]
            n303 = call "IMAQ Convert ROI to Line"("ROI Descriptor"=w275) -> ("Line"=w274:T16)  [unwired: 8 in, 1 out]
            n304 = call "IMAQ Centroid"("error in (no error)"=w267, "Image"=w256) -> ("error out"=w277:errorcluster, "Centroid"=→"Centroid":cluster{"X Centroid":sgl, "Y Centroid":sgl})  [unwired: 2 in]
            n305 = Unbundle(w274) -> ("Start X"=w273:i32, "Start Y"=w272:i32, "End X"=w271:i32, "End Y"=w270:i32)
            n306 = Build Array(w273, w272, w271, w270) -> (w269:i32[])
            n307 = call "IMAQ LineProfile"("error in (no error)"=w277, "Line Coordinates"=w269, "Image"=w256) -> ("error out"=w263:errorcluster, "Line Graph"=→"lineout":cluster{"x0":sgl, "dx":sgl, "Pixels Line":sgl[]})  [unwired: 2 in, 2 out]
            "analysis error" <- w263
            n308 = case shown="True" "LowPass" {
              tunnel: w256 -> [_ w282]
              tunnel: [w279 w284] -> w254
              tunnel: w255 -> [w279 w281]
              frame False {
              }
              frame True {
                n309 = call "IMAQ LowPass"("Image Src"=w282, "Size & Tolerance"="Size & Tolerance", "Image Dst"=w281) -> ("Image Dst Out"=w284:T6, "error out"=w280:errorcluster)  [unwired: 4 in]
                n310 = call <vilib>:"Clear Errors.vi"("error in (no error)"=w280) -> ()  [unwired: 6 in, 1 out]
              }
            }
            n311 = call "GetMaxCounts.vi"("New Image"=w254) -> ("Maximal Value"=w260:sgl, "Color"=w261:u32)
            "Max Counts" <- w260
            n312 = property on="Max Counts" class="Slide (strict)"("Fill Color"=w261) -> ()  [unwired: 2 in, 2 out]
            n313 = case shown="True" "beep if sat." {
              tunnel: w260 -> [_ w287]
              frame False {
              }
              frame True {
                n314 = Greater Or Equal?(x=w287, y="sat level") -> (x >= y?=w285:bool)
                n315 = case shown="True" w285 {
                  frame False {
                  }
                  frame True {
                    n316 = call <vilib>:"Beep.vi"() -> ()  [unwired: 12 in]
                  }
                }
              }
            }
            n317 = Divide(x=256.0, y=w260) -> (x/y=w264:dbl)
            n318 = case shown="True" "LowPass" {
              tunnel: w254 -> [w288 w289]
              tunnel: w264 -> [_ w292]
              tunnel: w263 -> [_ _]
              tunnel: [w288 w290] -> w257
              tunnel: w255 -> [_ _]
              frame False {
              }
              frame True {
                n319 = call "IMAQ Multiply"("Image Src A"=w289, "Constant"=w292, "Image Dst"=w289) -> ("Image Dst Out"=w290:T6, "error out"=w291:errorcluster)  [unwired: 4 in]
                n320 = call <vilib>:"Clear Errors.vi"("error in (no error)"=w291) -> ()  [unwired: 6 in, 1 out]
              }
            }
          }
        }
        "Image (IMAQ)" <- w202
        n321 = call "IMAQ GetImageSize"("Image"=w202, "error in (no error)"=w203) -> ("Y Resolution"=→"Y Resolution":i32, "X Resolution"=→"X Resolution":i32, "error out"=w204:errorcluster)  [unwired: 2 in]
        n322 = call <vilib>:"Clear Errors.vi"("error in (no error)"=w204) -> ()  [unwired: 6 in, 1 out]
        n323 = Not Equal?(x="Color table", y=w195) -> (x != y?=w194:bool)
        n324 = control-ref of="error (h)"() -> (w234:refnum<vi>)
        n325 = control-ref of="error message"() -> (w241:refnum<vi>)
        n326 = Not(x="resize") -> (.not. x?=w229:bool)
        n327 = Preview Queue Element ("get stop queue value")(queue=w213, timeout in ms (-1)=5) -> (queue out=w212:refnum<queue>, element=w210:bool)  [unwired: 1 in, 2 out]
        n328 = Or(x=w211, y=w210) -> (x .or. y?=w209:bool)
        n329 = case shown="True" w194 {
          tunnel: [w248 w249] -> w196
          tunnel: "Color table" -> [w248 w249]
          frame False {
          }
          frame True {
            w251 = u32 5 items=["Grayscale", "Binary", "Gradient", "Rainbow", "Temperature", "User Defined"] ("Palette:Palette Type")
            n330 = call "IMAQ color table presets.vi"("Color table"=w249) -> ("Array"=w250:cluster{"R":u8, "G":u8, "B":u8}[])  [unwired: 9 in, 1 out]
            n331 = property on="Image (IMAQ)" class="ImageControl"("Palette Type"=w251, "User Palette"=w250) -> ()  [unwired: 2 in, 2 out]
          }
        }
        n332 = And(x=w229, y=w228) -> (x .and. y?=w227:bool)
        n333 = case shown="True" w209 {
          selector: w209 -> [_ w308]
          frame False {
          }
          frame True {
            n334 = call "StopFGV.vi"("Command"=enum16{"set", "get", "init"}."set", "Stop"=w308) -> ()  [unwired: 8 in, 2 out]
          }
        }
        n335 = Select(t=w238, s=w235, f=w236) -> (s? t:f=w237:i32[])
        n336 = call "clearErrorMessageGUI.vi"("millisecond timer value"=w242, "Boolean"=w240, "error message"=w241, "reference"=w234) -> ("millisecond timer value 2"=w243:u32)
        n337 = case shown="True" w227 {
          selector: w227 -> [w304 w306]
          tunnel: [w304 FALSE] -> w231
          frame False {
          }
          frame True {
            n338 = control-ref of="resize"() -> (w307:refnum<vi>)
            n339 = property class="Bool (strict)"(reference=w307, "Val(Sgnl)"=w306) -> ()  [unwired: 1 in, 2 out]
          }
        }
      }
      n340 = Call Chain() -> (call chain=w117:string[])
      n341 = Array Size(array=w117) -> (size(s)=w133:i32)
      n342 = Decrement(x=w133) -> (x-1=w132:i32)
      n343 = call "preset SQL Queries.vi"("Preset Query"=Preset_Query_Enum."GetItemLocatorIP") -> ("error out"=w127:errorcluster, "data"=w121:string[][])  [unwired: 8 in, 1 out]
      n344 = Random Number (0-1)() -> (number: 0 to 1=w112:dbl)
      n345 = Index Array(array=w117, index=w132) -> (element=w131:string)
      n346 = Number To Fractional String(number=w112) -> (F-format string=w110:string)  [unwired: 3 in]
      n347 = Index Array(array=w121, index (row) #1=w124, index (col) #1=0 ("disabled index (col)"), index (row) #2=w124, index (col) #2=1 ("disabled index (col)")) -> (element #1=w119:string, element #2=w120:string)
      n348 = Decimal String To Number(string=w120) -> (number=w126:i32)  [unwired: 2 in, 1 out]
      n349 = Match Pattern(string=w131, regular expression=".vi") -> (before substring=w129:string)  [unwired: 1 in, 3 out]
      n350 = To Unsigned Word Integer(number=w126) -> (unsigned 16bit integer=w125:u16)
      n351 = Concatenate Strings(w129, w110) -> (w111:string)
      n352 = call "TCP Write Alive 2.vi"("MultiCast Port"=w125, "Stopqueue"=w118, "address"=w119, "Name"=w111, "error in (no error)"=w127) -> ("error out"=w116:errorcluster)  [unwired: 8 in, 2 out]
      n353 = call "IMAQ Dispose"("Image"=w191) -> ()  [unwired: 5 in, 1 out]
      n354 = call "EventsFGV.vi"("Command"=enum16{"get", "init"}."get") -> ("New Event"=w157:T13)  [unwired: 9 in, 1 out]
      n355 = Unregister For Events(event registration refnum=w161, error in=w159) -> (error out=w160:errorcluster)
      n356 = Destroy User Event(user event=w157, error in=w160) -> (error out=w114:errorcluster)
      n357 = call <vilib>:"Clear Errors.vi"("error in (no error)"=w114) -> ("error out"=w113:errorcluster)  [unwired: 6 in]
      n358 = Lossy Enqueue Element(queue=w118, element=w115, error in (no error)=w113) -> (error out=w141:errorcluster)  [unwired: 3 out]
      n359 = call <vilib>:"Clear Errors.vi"("error in (no error)"=w141) -> ("error out"=w140:errorcluster)  [unwired: 6 in]
      n360 = Merge Errors(w140, w116) -> (w136:errorcluster)
      n361 = Flush Queue(queue=w118, error in (no error)=w136) -> (queue out=w134:refnum<queue>, error out=w139:errorcluster)  [unwired: 1 out]
      n362 = local read "connections (hidden)"() -> (w186:variant[])
      n363 = Release Queue(queue=w134, force destroy? (F)=TRUE, error in (no error)=w139) -> (error out=w137:errorcluster)  [unwired: 2 out]
      n364 = call <vilib>:"Clear Errors.vi"("error in (no error)"=w137) -> ("error out"=w135:errorcluster)  [unwired: 6 in]
      n365 = call "Close UDP AND TCP connections.vi"("error in"=w135, "appended array"=w186) -> ()  [unwired: 6 in]
    }
    frame #4 {
      n366 = flat-sequence {
        frame #0 {
          n367 = Wait (ms)(milliseconds to wait=u32 0) -> ()  [unwired: 1 out]
        }
        frame #1 {
          n368 = local write "stop"(FALSE ("stop")) -> ()
        }
        frame #2 {
          n369 = disable-structure shown="Disabled" {
            frame Disabled {
              n370 = control-ref of="This VI"() -> (w566:refnum<vi>)
              n371 = case shown="False" FALSE {
                tunnel: w566 -> [w567 w570]
                tunnel: [w567 w568] -> w565
                frame False {
                }
                frame True {
                  n372 = property class="VI" props=["Front Panel.Open"](reference=w570) -> (reference out=w569:refnum<vi>)  [unwired: 1 in, 2 out]
                  n373 = invoke class="VI" method="FP.Close"(reference=w569) -> (reference out=w568:refnum<vi>)  [unwired: 2 in, 2 out]
                }
              }
              n374 = Close Reference(reference=w565) -> ()  [unwired: 1 in, 1 out]
            }
            frame Enabled {
            }
          }
        }
      }
      n375 = control-ref of="Main  Control"() -> (w560:refnum<vi>)
      n376 = property class="TabCtl (strict)"(reference=w560, "Tab Location"=enum32{"Top", "Bottom", "Left", "Right"}."Bottom") -> ()  [unwired: 1 in, 2 out]
      n377 = property class="TabCtl (strict)"(reference=w560, "Tabs Visible?"=TRUE) -> ()  [unwired: 1 in, 2 out]
    }
  }
  n378 = property on="Image (array)" class="IntGraph (strict)"("Color Table"=u32[] [16777215, 8126719, 7864574, 7536895, 7274750, 6947071, 6684926, 6357247, 6095102, 5767423, 5505278, 5177599, 4915454, 4587775, 4325630, 3997951, 3735806, 3408127, 3145982, 2818303, 2556158, 2228479, 1966334, 1638655, 1376510, 1048831, 786686, 459007, 196862, 767, 1790, 3071, 4094, 5375, 6398, 7679, 8702, 9983, 11006, 12287, 13310, 14591, 15614, 16895, 17918, 19199, 20222, 21503, 22526, 23807, 24830, 26111, 27134, 28415, 29438, 30719, 31486, 33023, 33790, 35327, 36094, 37631, 38398, 39935, 40702, 42239, 43006, 44543, 45310, 46847, 47614, 49151, 49918, 51455, 52222, 53759, 54526, 56063, 56830, 58367, 59134, 60671, 61694, 62975, 63998, 65279, 65274, 65527, 65265, 65518, 65256, 65509, 65247, 65500, 65238, 65491, 65229, 65482, 65220, 65473, 65211, 65464, 65202, 65455, 65193, 65446, 65184, 65437, 65175, 65428, 65166, 65419, 65157, 65410, 65149, 65401, 65140, 65392, 65131, 65383, 65122, 65374, 65113, 65365, 65104, 65356, 65095, 65347, 65086, 65338, 65077, 65329, 65068, 65320, 65059, 65311, 65050, 65302, 65041, 65293, 65032, 65284, 130560, 392960, 720384, 982784, 1310208, 1572608, 1900032, 2162432, 2489856, 2752256, 3079680, 3342080, 3669504, 3931904, 4259328, 4521728, 4849152, 5111552, 5438976, 5701376, 6028800, 6291200, 6618624, 6881024, 7208448, 7470848, 7798272, 8126208, 8322560, 8716032, 8912384, 9305856, 9502208, 9895680, 10092032, 10485504, 10681856, 11075328, 11271680, 11665152, 11861504, 12254976, 12451328, 12844800, 13041152, 13434624, 13630976, 14024448, 14220800, 14614272, 14810624, 15204096, 15400448, 15793920, 15990272, 16383744, 16580096, 16776192, 16709376, 16773888, 16707072, 16771584, 16704768, 16769280, 16702464, 16766976, 16700160, 16764672, 16697856, 16762368, 16695552, 16760064, 16693248, 16757760, 16690944, 16755456, 16688640, 16753152, 16686336, 16750848, 16684032, 16748544, 16681728, 16746240, 16679680, 16743936, 16677376, 16741632, 16675072, 16739328, 16672768, 16737024, 16670464, 16734720, 16668160, 16732416, 16665856, 16730112, 16663552, 16727808, 16661248, 16725504, 16658944, 16723200, 16656640, 16720896, 16654336, 16718592, 16652032, 16716288, 16649728, 16713984, 16712960, 0] ("256 rainbow")) -> ()  [unwired: 2 in, 2 out]
  n379 = control-ref of="This VI"() -> (w3:refnum<vi>)
  n380 = disable-structure "Factory Pattern: Enable plugin" shown="RUN_TIME_ENGINE==True" {
    disable-tunnel: w2 -> [_ w575]
    disable-tunnel: w3 -> [w571 w574]
    disable-tunnel: [_ w573] -> _
    disable-tunnel: [w571 w572] -> w1
    frame condition #0 (active) {
    }
    frame condition #1 {
      n381 = property class="VI"(reference=w574, error in=w575, "Front Panel.Open"=FALSE) -> (reference out=w572:refnum<vi>, error out=w573:errorcluster)
    }
  }
  n382 = Close Reference(reference=w1) -> ()  [unwired: 1 in, 1 out]
